vi "TestBench.subVI.GeneratePWM.vi"(8 "error in (no error)":errorcluster) -> (0 "error out":errorcluster, 2 "PWMs":dbl[][](array[numeric]))   [LabVIEW 2015]
uses:
  TestBenchVariables.vi
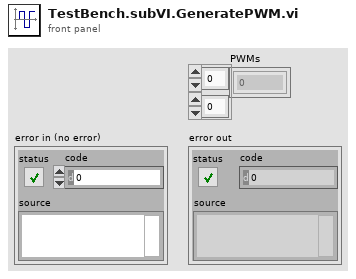
[diagram p1: front panel]
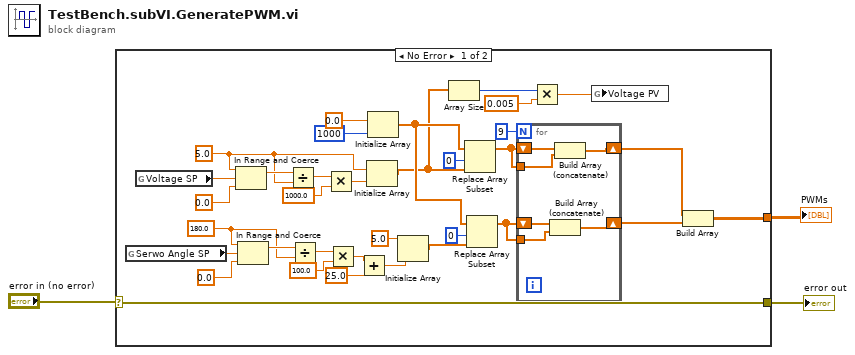
[diagram p0: block diagram]
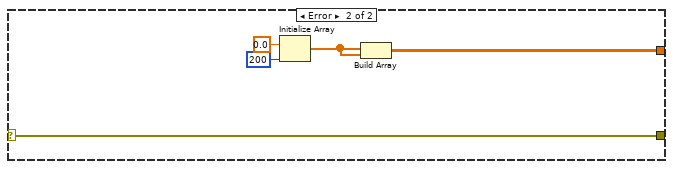
[diagram p2: hidden frame]
diagram:
  n1 = case shown="No Error" "error in (no error)" {
    selector: "error in (no error)" -> [w17 w44]
    tunnel: [w18 w45] -> w3
    tunnel: [w17 w44] -> w1
    frame No Error {
      w23 = 180.0 ("y")
      w30 = 5.0 ("y")
      n2 = global read "TestBenchVariables.vi" "Serwo Angle SP"() -> (w28:dbl)
      n3 = global read "TestBenchVariables.vi" "Voltage SP"() -> (w36:dbl)
      n4 = In Range and Coerce(upper limit=w30, x=w36, lower limit=0.0 ("y")) -> (coerced(x)=w34:dbl)  [unwired: 1 out]
      n5 = In Range and Coerce(upper limit=w23, x=w28, lower limit=0.0 ("y")) -> (coerced(x)=w26:dbl)  [unwired: 1 out]
      n6 = Divide(x=w34, y=w30) -> (x/y=w33:dbl)
      n7 = Divide(x=w26, y=w23) -> (x/y=w25:dbl)
      n8 = Multiply(x=w33, y=1000.0) -> (x*y=w31:dbl)
      n9 = Multiply(x=w25, y=100.0) -> (x*y=w16:dbl)
      n10 = Add(x=w16, y=25.0) -> (x+y=w14:dbl)
      n11 = Initialize Array(w30, w31) -> (w8:dbl[])
      n12 = Initialize Array(0.0 ("element"), 1000 ("dimension size")) -> (w19:dbl[])
      n13 = Initialize Array(5.0 ("element"), w14) -> (w22:dbl[])
      n14 = Array Size(array=w8) -> (size(s)=w6:i32)
      n15 = Replace Array Subset(array=w19, new element=w8, index=0) -> (w12:dbl[])
      n16 = Replace Array Subset(array=w19, new element=w22, index=0) -> (w11:dbl[])
      n17 = for {
        N: 9 -> [_]
        shift-right: [w42] -> w10
        shift-left: w12 -> [w43]
        tunnel: w12 -> [w41]
        shift-right: [w39] -> w9
        shift-left: w11 -> [w40]
        tunnel: w11 -> [w38]
        n18 = Build Array (concatenate)(w40, w38) -> (w39:dbl[])
        n19 = Build Array (concatenate)(w43, w41) -> (w42:dbl[])
      }
      n20 = Multiply(x=w6, y=0.005) -> (x*y=w4:dbl)
      n21 = global write "TestBenchVariables.vi" "Voltage PV"(w4) -> ()
      n22 = Build Array(w10, w9) -> (w18:dbl[][])
    }
    frame Error {
      n23 = Initialize Array(0.0 ("element"), 200 ("dimension size")) -> (w46:dbl[])
      n24 = Build Array(w46, w46) -> (w45:dbl[][])
    }
  }
  "PWMs" <- w3
  "error out" <- w1
